vi "libssh2_channel_wait_eof.vi"(8 "error in (no error)":errorcluster, 11 "channel":T1) -> (0 "error out":errorcluster)   [LabVIEW 2017, in "libssh2.lvlib"]
doc: "Wait for EOF on a channel."
uses:
  libssh2.lvlib
  Channel Refnum.ctl
  Acquire Session.vi
  Release Session.vi
  Not A Channel.vi
  <vilib>/Utility/error.llb/Error Cluster From Error Code.vi
  Global Settings.vi
  Read Channel Refnum.vi
  Read Session Refnum.vi
  <vilib>/Utility/semaphor.llb/Acquire Semaphore.vi
  <vilib>/Utility/semaphor.llb/Release Semaphore.vi
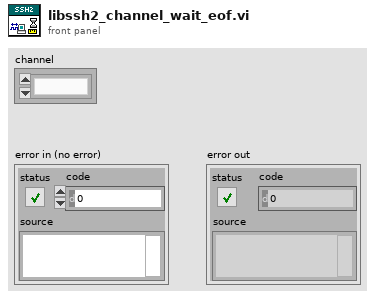
[diagram p1: front panel]
types:
  T1 = typedef "libssh2.lvlib/Channel Refnum.ctl" = refnum<k1>
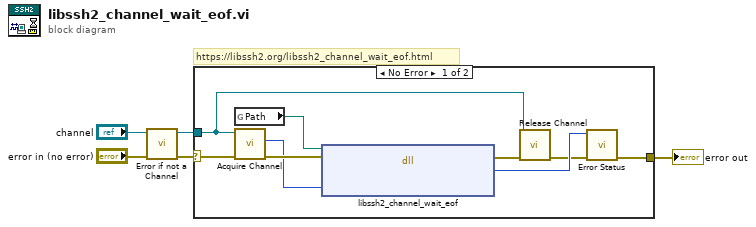
[diagram p0: block diagram]
diagram:
  # "https://libssh2.org/libssh2_channel_wait_eof.html"
  n1 = call "Error if not a Channel.vi"("error in (no error)"="error in (no error)", "channel"="channel") -> ("error out"=w3:errorcluster, "channel out"=w1:T1)  [unwired: 8 in]
  n2 = case shown="No Error" w3 {
    selector: w3 -> [w14 w15]
    tunnel: [w13 w15] -> w5
    tunnel: w1 -> [w6 _]
    frame No Error {
      n3 = global read "Global Settings.vi" "Path"() -> (w9:path)
      n4 = call "Acquire Channel.vi"("error in (no error)"=w14, "channel"=w6) -> ("error out"=w11:errorcluster, "LIBSSH2_CHANNEL*"=w10:u64)  [unwired: 8 in]
      n5 = dll-call lib="?" fn="libssh2_channel_wait_eof"(path in=w9, error in=w11, "channel"=w10) -> (error out=w12:errorcluster, "return value"=w8:i32)  [unwired: 2 in, 1 out]
      n6 = call "Release Channel.vi"("error in (no error)"=w12, "channel"=w6) -> ("error out"=w7:errorcluster)  [unwired: 9 in]
      n7 = call "Error Status.vi"("error in (no error)"=w7, "return value"=w8) -> ("error out"=w13:errorcluster)  [unwired: 8 in, 1 out]
    }
    frame Error {
    }
  }
  "error out" <- w5
